vi "Set Encoder UI from file.vi"(8 "error in (no error)":errorcluster, 11 "Encoder available":bool) -> (0 "error out":errorcluster)   [LabVIEW 2013]
uses:
  Typedefs/Which path.ctl
  Global Variables/gl_UI Ctrl Refs.vi
  <vilib>/Utility/config.llb/NI_LVConfig.lvlib
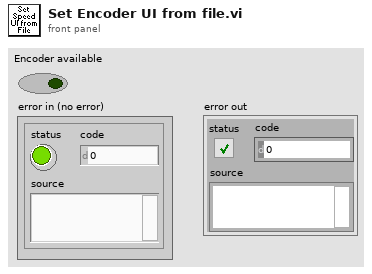
[diagram p1: front panel]
types:
  T1 = cluster{"key":string, "Save?":bool, "Default":bool}
  T2 = typedef "Which path.ctl" = enum16{"Configuration Files", "Calibration Files", "Images", "Setup.ini", "Loaded User profile.ini", "User's-Previous session.ini", "New user profile.ini", "Selected User profile.ini", "User profiles folder", "Power meter scaling.txt", "FOV Cal.ini"}
  T3 = typedef "NI_LVConfig.lvlib/Config Data RefNum.ctl" = refnum<k1>
  T4 = cluster{"key":string, "Save?":bool, "Default":bool}[]
  T5 = typedef "UI ctrl refs cluster.ctl" = cluster{"Top level VI path":path, "Top level VI ref":refnum<vi>, "User menu ref":refnum<k9>, "Sub Panel control":refnum<vi>, "Imaging Param Tab":refnum<vi>, "Occurrence-Start drivers":refnum<k4>, "Occurrence-Speed logging initialised":refnum<k4>, "Occurrence-XYZ stage initialised":refnum<k4>, "Exit button":refnum<vi>, "Status ind":refnum<vi>, "Return to Origin":refnum<vi>, "Speed Logging":refnum<vi>, "Time Lapse":refnum<vi>, "Live Imaging":refnum<vi>, "AOL Z Stack":refnum<vi>, "Motor Z Stack":refnum<vi>, "Funct Acq button":refnum<vi>, "Hard Shutter":refnum<vi>, "Virtual Shutter":refnum<vi>, "Laser Power":refnum<vi>, "AOL Mode":refnum<vi>, "Frame Size":refnum<vi>, "Field of View":refnum<vi>, "Dwell Time":refnum<vi>, "Zoom":refnum<vi>, "AOL Z":refnum<vi>, "Objective":refnum<vi>, "Axis":refnum<vi>, "Paths & Names":refnum<vi>, "Experiment folder path (ind.)":refnum<vi>, "Last State (Ind.)":refnum<vi>, "Laser wavelength ind (nm)":refnum<vi>, "Averages":refnum<vi>, "Angle (degrees)":refnum<vi>, "X centre":refnum<vi>, "Y centre":refnum<vi>, "Plane Mode":refnum<vi>, "# Planes":refnum<vi>, "Z Start":refnum<vi>, "Z Stop":refnum<vi>, "Z Step":refnum<vi>, "PMT 1":refnum<vi>, "PMT 2":refnum<vi>, "Stage XYZ Position":refnum<vi>, "Pockels@Z Start":refnum<vi>, "Pockels@Z Stop":refnum<vi>, "Obtain Z Start":refnum<vi>, "Obtain Z Stop":refnum<vi>, "Live stim.trig.period":refnum<vi>, "Live stim.trig.enable":refnum<vi>, "Funct. Acq. Pockels Modulation":refnum<vi>, "Enable Video Recording":refnum<vi>, "Video Record-Live Imaging":refnum<vi>, "Video Record-Funct acq":refnum<vi>, "AOL Z-stack Chirps Ready (ind)":refnum<vi>, "Center freq ind (nm)":refnum<vi>, "Logging queue (ind)":refnum<vi>, "Back aperture power (ind.)":refnum<vi>, "Power after objective (ind.)":refnum<vi>, "Switch user":refnum<vi>}
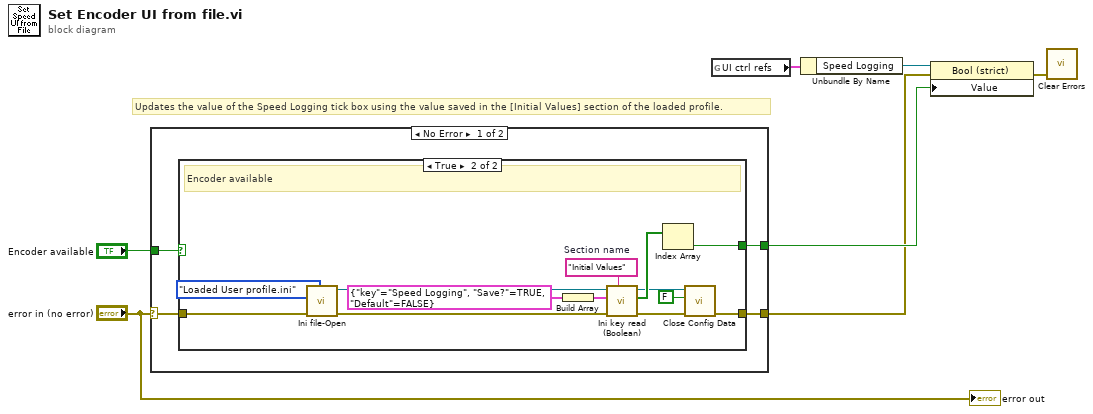
[diagram p0: block diagram]
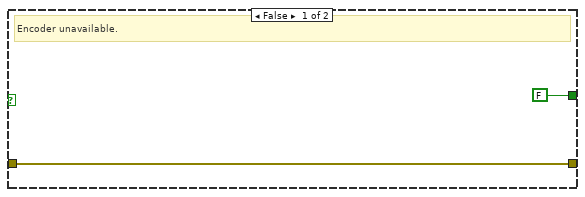
[diagram p2: hidden frame]
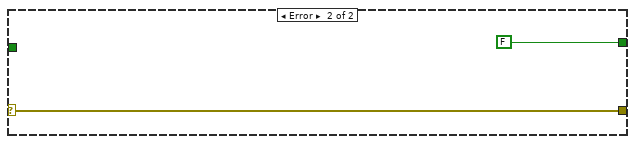
[diagram p3: hidden frame]
diagram:
  # "Updates the value of the Speed Logging tick box using the value saved in the [Initial Values] section of the loaded profile."
  n1 = case shown="No Error" "error in (no error)" {
    selector: "error in (no error)" -> [w11 w28]
    tunnel: [w10 w28] -> w2
    tunnel: "Encoder available" -> [w9 _]
    tunnel: [w8 FALSE ("value")] -> w3
    frame No Error {
      n2 = case shown="True" w9 {
        tunnel: w11 -> [w13 w16]
        tunnel: [w13 w14] -> w10
        tunnel: [FALSE ("value") w15] -> w8
        frame False {
          # "Encoder unavailable."
        }
        frame True {
          w21 = "Initial Values"  # Section name
          # "Encoder available"
          n3 = call "Ini file-Open.vi"("Error In"=w16, "Which file?"=Which_path."Loaded User profile.ini") -> ("error out"=w22:errorcluster, "User profile ini file ref"=w23:T3)  [unwired: 6 in, 2 out]
          n4 = Build Array(T1 {"key"="Speed Logging", "Save?"=TRUE, "Default"=FALSE}) -> (w24:T4)
          n5 = call "Ini key read (Boolean).vi"("Section"=w21, "error in (no error)"=w22, "Parameter names & setup"=w24, "Ini file refnum in"=w23) -> ("error out"=w17:errorcluster, "Value read/used"=w20:bool[], "Ini file refnum out"=w18:T3)  [unwired: 5 in]
          n6 = Index Array(array=w20) -> (element=w15:bool)  [unwired: 1 in]
          n7 = call <vilib>:"Close Config Data.vi"("error in (no error)"=w17, "write file if changed (T)"=FALSE ("write configuration file? (F)"), "refnum"=w18) -> ("error out"=w14:errorcluster)  [unwired: 7 in, 1 out]
        }
      }
    }
    frame Error {
    }
  }
  n8 = global read "gl_UI Ctrl Refs.vi" "UI ctrl refs"() -> (w5:T5)
  n9 = Unbundle By Name(w5) -> ("Speed Logging"=w4:refnum<vi>)
  n10 = property class="Bool (strict)"(reference=w4, error in=w2, "Value"=w3) -> (error out=w6:errorcluster)  [unwired: 1 out]
  n11 = call <vilib>:"Clear Errors.vi"("error in (no error)"=w6) -> ()  [unwired: 6 in, 1 out]
  "error out" <- "error in (no error)"
